vi "SoundInputFFTOutput.vi"() -> (2 "dt":dbl, 3 "FFT {X}":cdb[](array[numeric]))   [LabVIEW 2014]
uses:
  <vilib>/Analysis/2dsp.llb/Real FFT.vi
  <vilib>/Analysis/NI_AALPro.lvlib
panel:
  out "1/x":dbl
  out "size(s) 2":i32[](array[numeric])
  out "FFT {X} 2":cdb[][](array[numeric])
  out "size(s)":i32
  in  "Path":path=path "U:/phys 434/Project/WeSawTheGoal.WAV"
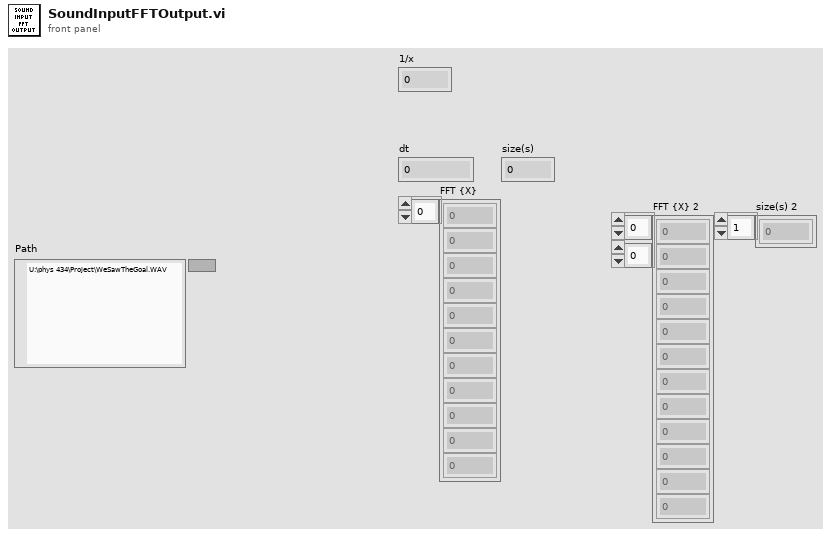
[diagram p1: front panel]
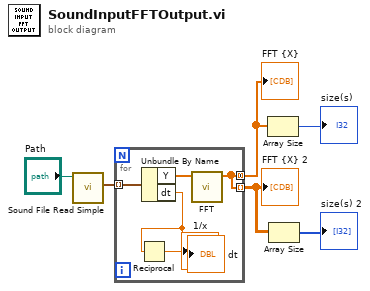
[diagram p0: block diagram]
diagram:
  n1 = call <vilib>:"Sound File Read Simple.vi"("path"="Path") -> ("data"=w3:waveform(dbl)[])  [unwired: 7 in, 3 out]
  n2 = for {
    tunnel: w3 -> [w11] mode=indexing
    tunnel: [w9] -> w6 mode=concatenating
    tunnel: [w9] -> w2 mode=indexing
    n3 = Unbundle By Name(w11) -> ("Y"=w10:dbl[], "dt"=w8:dbl)
    "dt" <- w8
    n4 = Reciprocal(x=w8) -> (1/x=→"1/x":dbl)
    n5 = call-poly <vilib>:"FFT.vi"("X"=w10) -> ("FFT {X}"=w9:cdb[])  [unwired: 9 in, 1 out]
  }
  "FFT {X}" <- w6
  "FFT {X} 2" <- w2
  n6 = Array Size(array=w6) -> (size(s)=→"size(s)":i32)
  n7 = Array Size(array=w2) -> (size(s)=→"size(s) 2":i32[])
